vi "Serialize to JSON.vi"(8 "error in (no error)":errorcluster, 11 "Package in":refnum<class "Package.lvclass">) -> (0 "error out":errorcluster, 1 "JSON Value":refnum<class "JSON Value.lvclass">, 2 "JSON string":string, 3 "Package out":refnum<class "Package.lvclass">)   [LabVIEW 2016, in "Packages.lvlib" / "Package.lvclass"]
uses:
  Package.lvclass
  <vilib>/addons/JSON API/JSON Value/JSON Value.lvclass
  Package.lvclass/Package.ctl
  <vilib>/addons/JSON API/JSON Array/JSON Array.lvclass
  C:/Program Files (x86)/National Instruments/LabVIEW 2016/vi.lib/addons/JSON API/JSON Value/JSON Value.lvclass
  Package Version_class/Package Version.lvclass
  <vilib>/addons/JSON API/Variant JSON/Variant JSON.lvlib
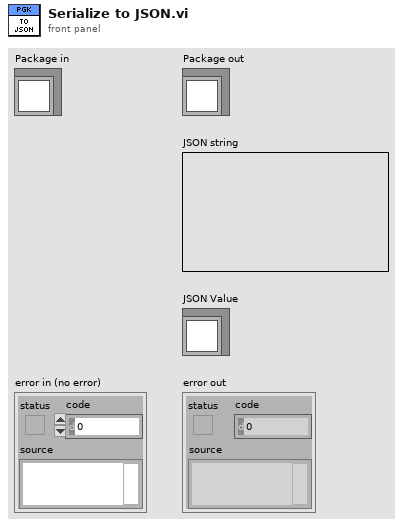
[diagram p1: front panel]
types:
  T1 = typedef "Packages.lvlib/Repo.lvclass/RepoType--enum.ctl" = enum16{"VIPM", "NIPM", "GPM"}
  T2 = cluster{"Name":string, "DisplayName":string, "RepoType":T1, "RepoName":string}
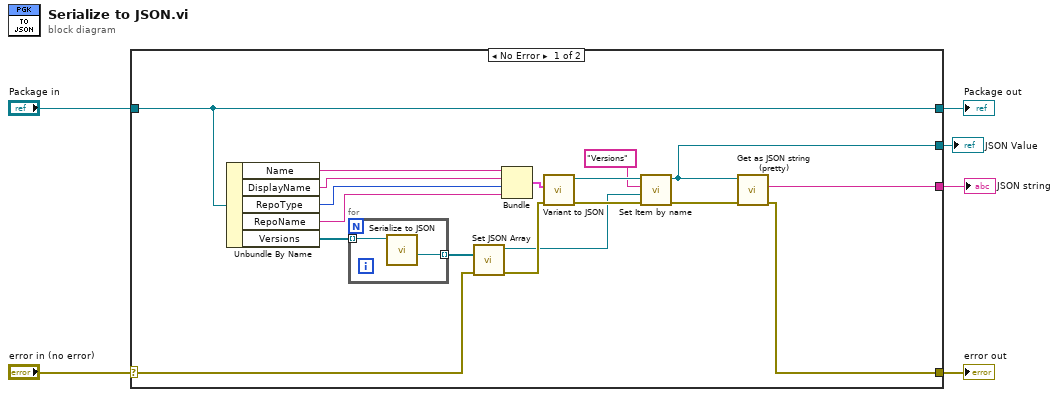
[diagram p0: block diagram]
diagram:
  n1 = case shown="No Error" "error in (no error)" {
    selector: "error in (no error)" -> [w18 w28]
    tunnel: [w17 w28] -> w5
    tunnel: [w24 w27] -> w3
    tunnel: "Package in" -> [w24 w27]
    tunnel: [w19 _] -> w2
    tunnel: [w12 _] -> w1
    frame No Error {
      n2 = Unbundle By Name(w24) -> ("Name"=w23:string, "DisplayName"=w22:string, "RepoType"=w21:T1, "RepoName"=w7:string, "Versions"=w15:refnum<class "Package Version.lvclass">[])
      n3 = for {
        tunnel: w15 -> [w26] mode=indexing
        tunnel: [w25] -> w10 mode=indexing
        n4 = call-dynamic "Serialize to JSON.vi"("Pkg Details in"=w26) -> ("JSON Value"=w25:refnum<class "JSON Value.lvclass">)  [unwired: 7 in, 3 out]
      }
      n5 = call <vilib>:"Set JSON Array.vi"("error in (no error)"=w18, "Array"=w10) -> ("error out"=w11:errorcluster, "JSON Array out"=w9:refnum<class "JSON Array.lvclass">)  [unwired: 8 in]
      n6 = Bundle("Name"=w23, "DisplayName"=w22, "RepoType"=w21, "RepoName"=w7) -> (w16:T2)  [unwired: 1 in]
      n7 = call <vilib>:"Variant to JSON.vi"("error in (no error)"=w11, "Variant"=w16) -> ("error out"=w20:errorcluster, "JSON Value out"=w13:refnum<class "JSON Value.lvclass">)  [unwired: 8 in]
      n8 = call-dynamic "Set Item by name.vi"("error in (no error)"=w20, "Value"=w9, "name"="Versions", "JSON Value In"=w13) -> ("error out"=w14:errorcluster, "JSON Value Out"=w12:refnum<class "JSON Value.lvclass">)  [unwired: 5 in, 1 out]
      n9 = call <vilib>:"Get as JSON string (pretty).vi"("error in (no error)"=w14, "JSON Value in"=w12) -> ("error out"=w17:errorcluster, "<JSON>"=w19:string)  [unwired: 8 in]
    }
    frame Error {
    }
  }
  "error out" <- w5
  "Package out" <- w3
  "JSON string" <- w2
  "JSON Value" <- w1
